vi "clean up plot.vi"() -> ()   [LabVIEW 2025]
panel:
  in  "y":dbl(slide) scale=0.0..2.0
  in  "XY Graph 3":cluster{"X":dbl, "Y":dbl}[](graph)=[{"X"=0.0, "Y"=3.7}, {"X"=0.05545055555555556, "Y"=3.9}, {"X"=0.07381444444444445, "Y"=4.0}, {"X"=0.09217861111111111, "Y"=4.0}, {"X"=0.11054305555555555, "Y"=4.0}, {"X"=0.1289072222222222, "Y"=4.0}, {"X"=0.14727166666666666, "Y"=4.0}, {"X"=0.16563583333333334, "Y"=4.0}, {"X"=0.184, "Y"=4.0}, {"X"=0.20236444444444443, "Y"=4.0}, {"X"=0.22072861111111114, "Y"=4.0}, {"X"=0.23909305555555557, "Y"=4.0}, {"X"=0.2574572222222222, "Y"=4.0}, {"X"=0.27582138888888885, "Y"=4.1}, {"X"=0.2941858333333333, "Y"=4.2}, {"X"=0.31255, "Y"=4.3}, {"X"=0.33091444444444446, "Y"=4.4}, {"X"=0.34927861111111114, "Y"=4.5}, {"X"=0.3676430555555556, "Y"=4.6}, {"X"=0.3860072222222222, "Y"=4.7}, {"X"=0.40437138888888896, "Y"=4.8}, {"X"=0.4227358333333333, "Y"=5.0}, {"X"=0.4411002777777778, "Y"=5.0}, {"X"=0.4594644444444444, "Y"=5.0}, {"X"=0.4778286111111111, "Y"=5.0}, {"X"=0.4961930555555556, "Y"=5.0}, {"X"=0.5145572222222222, "Y"=5.0}, {"X"=0.5329219444444445, "Y"=5.0}, {"X"=0.5512855555555555, "Y"=5.0}, {"X"=0.5696508333333333, "Y"=5.0}, {"X"=0.5880147222222223, "Y"=5.0}, {"X"=0.6063786111111111, "Y"=5.0}, {"X"=0.6247427777777778, "Y"=5.0}, {"X"=0.6431069444444444, "Y"=5.0}, {"X"=0.6614713888888889, "Y"=5.0}, {"X"=0.6798355555555555, "Y"=5.0}, {"X"=0.7349286111111112, "Y"=5.0}, {"X"=0.7805333333333333, "Y"=5.0}, {"X"=0.7988966666666666, "Y"=5.0}, {"X"=0.8172608333333334, "Y"=5.1}, {"X"=0.8356250000000001, "Y"=5.2}, {"X"=0.8539891666666666, "Y"=5.3}, {"X"=0.8723550000000001, "Y"=5.4}, {"X"=0.8907177777777778, "Y"=5.5}, {"X"=0.9090819444444446, "Y"=5.6}, {"X"=0.9274463888888889, "Y"=5.7}, {"X"=0.9458105555555556, "Y"=5.8}, {"X"=0.9641755555555557, "Y"=6.0}, {"X"=0.9825413888888889, "Y"=6.0}, {"X"=1.0009066666666666, "Y"=6.0}, {"X"=1.0192705555555555, "Y"=6.0}, {"X"=1.0376347222222224, "Y"=6.1}, {"X"=1.0559997222222224, "Y"=6.2}, {"X"=1.0743633333333333, "Y"=6.3}, {"X"=1.0927274999999999, "Y"=6.4}, {"X"=1.1110919444444443, "Y"=6.6}, {"X"=1.129456111111111, "Y"=6.7}, {"X"=1.1478205555555556, "Y"=6.8}, {"X"=1.1661861111111114, "Y"=7.0}, {"X"=1.1845522222222222, "Y"=7.1}, {"X"=1.2029188888888889, "Y"=7.3}, {"X"=1.2212858333333332, "Y"=7.4}, {"X"=1.23965, "Y"=7.6}, {"X"=1.2580144444444445, "Y"=7.8}, {"X"=1.2763786111111108, "Y"=7.9}, {"X"=1.294743888888889, "Y"=8.2}, {"X"=1.3131072222222222, "Y"=8.4}, {"X"=1.3314713888888887, "Y"=8.6}, {"X"=1.3498358333333333, "Y"=8.8}, {"X"=1.3682002777777778, "Y"=9.1}, {"X"=1.3865644444444445, "Y"=9.3}, {"X"=1.4049286111111112, "Y"=9.6}, {"X"=1.4232947222222223, "Y"=9.8}, {"X"=1.44166, "Y"=10.1}, {"X"=1.460024166666667, "Y"=10.4}, {"X"=1.478388888888889, "Y"=10.7}, {"X"=1.496752777777778, "Y"=11.0}, {"X"=1.5151172222222222, "Y"=11.4}, {"X"=1.533481388888889, "Y"=11.7}, {"X"=1.5518455555555557, "Y"=12.0}, {"X"=1.57021, "Y"=12.4}, {"X"=1.5885741666666668, "Y"=12.7}, {"X"=1.6069383333333334, "Y"=13.1}, {"X"=1.625302777777778, "Y"=13.5}, {"X"=1.6436669444444445, "Y"=13.9}, {"X"=1.662031388888889, "Y"=14.2}, {"X"=1.6987597222222222, "Y"=14.6}, {"X"=1.7171241666666668, "Y"=15.5}, {"X"=1.7905811111111112, "Y"=15.9}, {"X"=1.8089455555555556, "Y"=17.6}, {"X"=1.827309722222222, "Y"=18.1}, {"X"=1.8456741666666665, "Y"=18.6}, {"X"=1.8640386111111111, "Y"=19.0}, {"X"=1.8824025000000002, "Y"=19.5}, {"X"=1.9007669444444446, "Y"=20.0}, {"X"=1.9191311111111111, "Y"=20.4}, {"X"=1.9374952777777779, "Y"=20.9}, {"X"=1.9558608333333334, "Y"=21.4}, {"X"=1.974223888888889, "Y"=21.9}, {"X"=1.9925883333333334, "Y"=22.4}, {"X"=2.010952777777778, "Y"=22.9}, {"X"=2.029317222222222, "Y"=23.5}, {"X"=2.0476811111111113, "Y"=24.0}, {"X"=2.0660499999999997, "Y"=24.5}, {"X"=2.0844150000000004, "Y"=25.1}, {"X"=2.1027794444444448, "Y"=25.7}, {"X"=2.121143888888889, "Y"=26.2}, {"X"=2.1395080555555555, "Y"=26.8}, {"X"=2.157872222222222, "Y"=27.4}, {"X"=2.176236388888889, "Y"=28.0}, {"X"=2.1946008333333333, "Y"=28.6}, {"X"=2.2129649999999996, "Y"=29.2}, {"X"=2.231329444444444, "Y"=29.8}, {"X"=2.249693611111111, "Y"=30.4}, {"X"=2.2680577777777775, "Y"=31.1}, {"X"=2.2864225, "Y"=31.7}, {"X"=2.3047863888888886, "Y"=32.3}, {"X"=2.323150833333334, "Y"=33.0}, {"X"=2.341515, "Y"=33.7}, {"X"=2.3598791666666665, "Y"=34.3}, {"X"=2.378243611111111, "Y"=35.0}, {"X"=2.396608055555556, "Y"=35.7}, {"X"=2.4149722222222225, "Y"=36.4}, {"X"=2.4333363888888893, "Y"=37.1}, {"X"=2.451700833333333, "Y"=37.8}, {"X"=2.470065, "Y"=38.5}, {"X"=2.4884291666666667, "Y"=39.2}, {"X"=2.5067936111111115, "Y"=39.9}, {"X"=2.525157777777778, "Y"=40.6}, {"X"=2.543522777777778, "Y"=41.4}, {"X"=2.5618863888888885, "Y"=42.1}, {"X"=2.580251388888889, "Y"=42.8}, {"X"=2.8740788888888886, "Y"=54.4}, {"X"=2.8924433333333335, "Y"=55.1}, {"X"=2.9108077777777774, "Y"=55.8}, {"X"=2.929171944444444, "Y"=56.5}, {"X"=2.947536111111111, "Y"=57.2}, {"X"=2.9659002777777776, "Y"=57.9}, {"X"=2.984264722222222, "Y"=58.6}, {"X"=3.002628888888889, "Y"=59.3}, {"X"=3.020993055555556, "Y"=60.0}, {"X"=3.0393575, "Y"=60.7}, {"X"=3.0577224999999997, "Y"=61.3}, {"X"=3.076086944444445, "Y"=62.0}, {"X"=3.0944502777777783, "Y"=62.8}, {"X"=3.1128144444444446, "Y"=63.5}, {"X"=3.131178888888889, "Y"=64.2}, {"X"=3.1495430555555552, "Y"=64.9}, {"X"=3.1679077777777778, "Y"=65.6}, {"X"=3.186271666666667, "Y"=66.3}, {"X"=3.2046361111111112, "Y"=67.0}, {"X"=3.2230005555555556, "Y"=67.7}, {"X"=3.2413644444444443, "Y"=68.4}, {"X"=3.2597288888888887, "Y"=69.1}, {"X"=3.278093055555556, "Y"=69.8}, {"X"=3.296457222222222, "Y"=70.5}, {"X"=3.3148216666666666, "Y"=71.1}, {"X"=3.333185833333333, "Y"=71.8}, {"X"=3.3515502777777777, "Y"=72.5}, {"X"=3.3699149999999998, "Y"=73.1}, {"X"=3.388278611111111, "Y"=73.8}, {"X"=3.4066430555555556, "Y"=74.4}, {"X"=3.4250075, "Y"=75.0}, {"X"=3.4433716666666667, "Y"=75.6}, {"X"=3.461736388888889, "Y"=76.2}, {"X"=3.4801, "Y"=76.8}, {"X"=3.4984650000000004, "Y"=77.4}, {"X"=3.516828611111111, "Y"=78.0}, {"X"=3.5351930555555553, "Y"=78.6}, {"X"=3.5535572222222225, "Y"=79.1}, {"X"=3.5719213888888888, "Y"=79.7}, {"X"=3.5902858333333336, "Y"=80.3}, {"X"=3.6086508333333334, "Y"=80.8}, {"X"=3.6270147222222224, "Y"=81.4}, {"X"=3.6453791666666664, "Y"=81.9}, {"X"=3.663742777777778, "Y"=82.5}, {"X"=3.682107222222222, "Y"=83.0}, {"X"=3.7004719444444447, "Y"=83.6}, {"X"=3.718835833333333, "Y"=84.1}, {"X"=3.7372005555555554, "Y"=84.6}, {"X"=3.755564166666667, "Y"=85.2}, {"X"=3.773928611111111, "Y"=85.7}, {"X"=3.792293055555555, "Y"=86.2}, {"X"=3.8106569444444447, "Y"=86.7}, {"X"=3.8290233333333332, "Y"=87.3}, {"X"=3.8473888888888887, "Y"=87.8}, {"X"=3.865752777777778, "Y"=88.3}, {"X"=3.884117222222222, "Y"=88.9}, {"X"=3.9024811111111117, "Y"=89.4}, {"X"=3.920846111111111, "Y"=90.0}, {"X"=3.9392097222222224, "Y"=90.5}, {"X"=3.957574166666667, "Y"=91.0}, {"X"=3.9759383333333336, "Y"=91.4}, {"X"=3.9943027777777775, "Y"=91.9}, {"X"=4.0126675, "Y"=92.3}, {"X"=4.031031666666666, "Y"=92.7}, {"X"=4.049395555555556, "Y"=93.1}, {"X"=4.067759722222222, "Y"=93.5}, {"X"=4.086123888888889, "Y"=93.9}, {"X"=4.104488888888889, "Y"=94.3}, {"X"=4.122852777777778, "Y"=94.6}, {"X"=4.141216666666667, "Y"=94.9}, {"X"=4.159581111111112, "Y"=95.2}, {"X"=4.177945277777778, "Y"=95.5}, {"X"=4.196309722222222, "Y"=95.8}, {"X"=4.214684166666666, "Y"=96.1}, {"X"=4.233050277777777, "Y"=96.3}, {"X"=4.269777777777778, "Y"=96.5}, {"X"=4.288142222222222, "Y"=96.9}, {"X"=4.306506944444445, "Y"=97.0}, {"X"=4.324871111111111, "Y"=97.1}, {"X"=4.343235000000001, "Y"=97.3}, {"X"=4.361599166666666, "Y"=97.4}, {"X"=4.379963333333333, "Y"=97.5}, {"X"=4.398327777777777, "Y"=97.6}, {"X"=4.416692222222222, "Y"=97.8}, {"X"=4.435056388888889, "Y"=97.9}, {"X"=4.453420555555556, "Y"=98.0}, {"X"=4.471784722222222, "Y"=98.0}, {"X"=4.490149166666667, "Y"=98.0}, {"X"=4.508513333333332, "Y"=98.0}, {"X"=4.526877499999999, "Y"=98.0}, {"X"=4.545241944444444, "Y"=98.0}, {"X"=4.563606666666667, "Y"=98.0}, {"X"=4.581970555555556, "Y"=98.0}, {"X"=4.6003347222222235, "Y"=98.0}, {"X"=4.618699166666667, "Y"=98.0}, {"X"=4.637063333333333, "Y"=98.0}, {"X"=4.6554275, "Y"=98.0}, {"X"=4.673791666666667, "Y"=98.0}, {"X"=4.692156111111111, "Y"=98.0}, {"X"=4.7105202777777775, "Y"=98.0}, {"X"=4.728884722222222, "Y"=98.0}, {"X"=4.7472488888888895, "Y"=98.0}, {"X"=4.765613055555556, "Y"=98.0}, {"X"=4.783977777777777, "Y"=98.0}, {"X"=4.802341666666667, "Y"=98.0}, {"X"=4.820705833333334, "Y"=98.0}, {"X"=4.839070277777777, "Y"=98.0}, {"X"=4.857434444444444, "Y"=98.0}, {"X"=4.875798888888889, "Y"=98.0}, {"X"=4.894163333333334, "Y"=98.0}]
  out "index":i32(slide) scale=0.0..10000000.0
  out "XY Graph 2":T1(graph)
  in  "XY Graph":cluster{"X":dbl, "Y":dbl}[](graph)
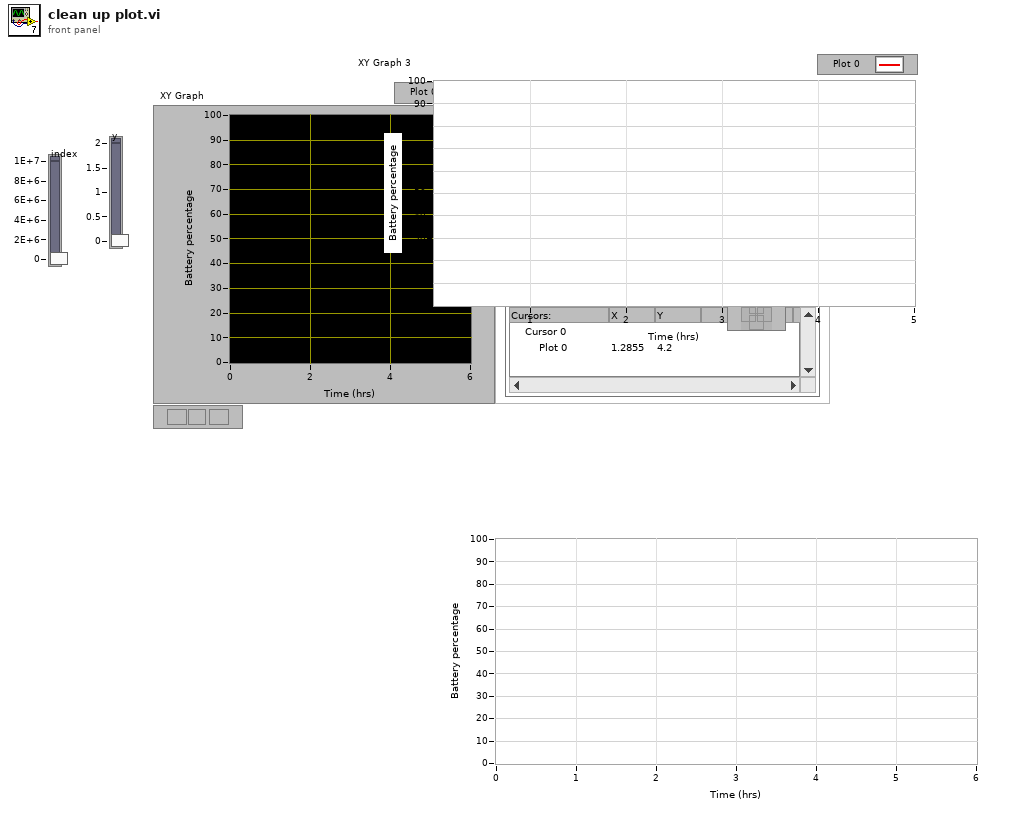
[diagram p1: front panel]
types:
  T1 = cluster{"XY Graph":cluster{"X":dbl, "Y":dbl}[]}[]
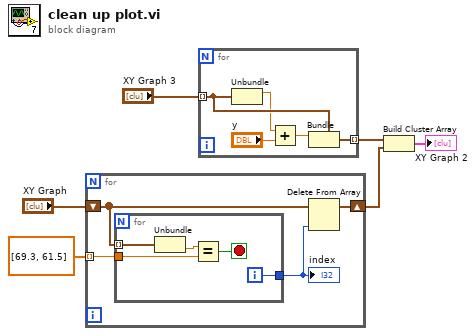
[diagram p0: block diagram]
diagram:
  n1 = for {
    tunnel: dbl[] [69.3, 61.5] -> [w7] mode=indexing
    shift-right: [w10] -> w3
    shift-left: "XY Graph" -> [w9]
    n2 = for {
      tunnel: w9 -> [w15] mode=indexing
      tunnel: [w12] -> w8
      tunnel: w7 -> [w11]
      i -> [w12]
      stop <- w13 stop-if-true
      n3 = Unbundle(w15) -> ("Y"=w14:dbl)  [unwired: 1 out]
      n4 = Equal?(x=w14, y=w11) -> (x = y?=w13:bool)
    }
    "index" <- w8
    n5 = Delete From Array(array=w9, index=w8) -> (array with subset deleted=w10:cluster{"X":dbl, "Y":dbl}[])  [unwired: 1 in, 1 out]
  }
  n6 = for {
    tunnel: "XY Graph 3" -> [w20] mode=indexing
    tunnel: [w19] -> w1 mode=indexing
    n7 = Unbundle(w20) -> ("X"=w18:dbl)  [unwired: 1 out]
    n8 = Add(x=w18, y="y") -> (x+y=w17:dbl)
    n9 = Bundle(cluster=w20, "X"=w17) -> (w19:cluster{"X":dbl, "Y":dbl})  [unwired: 1 in]
  }
  n10 = Build Cluster Array(w1, w3) -> (→"XY Graph 2":T1)
